vi "ni5660 Configure for IQ.vi"(0 "receiver info in":T1, 1 "acquisition type":string(combo)="FINITE", 5 "carrier frequency (Hz)":dbl=100000000.0 format="%.2p", 7 "bandwidth (Hz)":dbl=20000000.0 format="%.2p", 9 "time duration (sec)":dbl=1e-05 format="%.2p", 11 "error in (no error)":errorcluster, 12 "reference level (dBm)":i32, 13 "auto attenuation":enum16{"DISABLE", "ENABLE"}(ring)=enum."ENABLE", 14 "attenuation (dB)":i32=20) -> (4 "receiver info out":T1, 15 "error out":errorcluster)   [LabVIEW 2011]
doc: "This VI configures the RF Signal Analyzer hardware to acquire a time-domain signal with IQ settings you specify. Carrier frequency, bandwidth, and acquisition time settings define the IQ data. You can configure the acquisition to be finite or continuous. \n\nThis VI configures the reference level and attenuation settings used by the RF downconverter module, and the horizontal settings and acquisition type used by the IF digitizer module."
uses:
  <vilib>/addons/Modulation/niScope/controls/mod_Modulation Settings.ctl
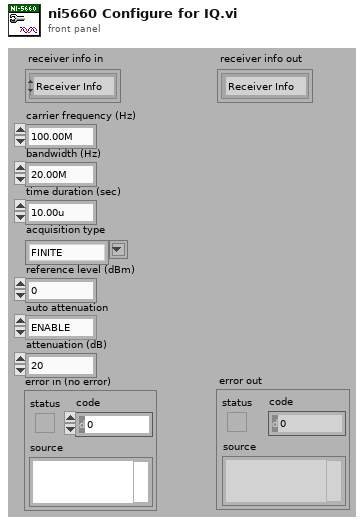
[diagram p1: front panel]
types:
  T1 = typedef "mod_Modulation Settings.ctl" = cluster{enum16{"Receiver Info"}, variant}
  T2 = typedef "mod_Readable Attributes Cluster.ctl" = cluster{"carrier":cluster{"frequency":dbl}, "receiver":cluster{"handles":cluster{"niTuner taskID":i32, "niScope handle":refnum<k15>}, "RFSA":cluster{"reference level":i32, "RF attenuation":i32}, "data format":enum16{"real", "complex modulated (array)", "complex modulated (interleaved)"}, "auto suppress SW IQ":enum16{"off", "on"}, "IQ sample rate":dbl, "bandwidth":dbl}}
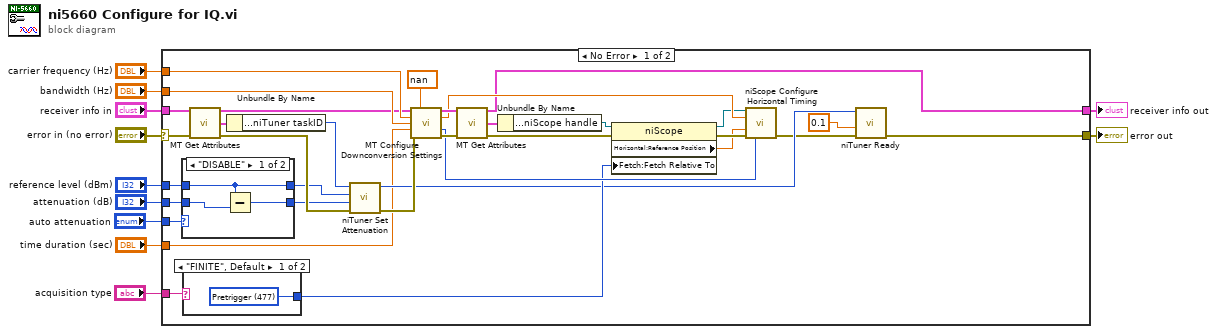
[diagram p0: block diagram]
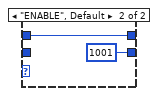
[diagram p2: hidden frame]
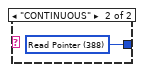
[diagram p3: hidden frame]
diagram:
  n1 = case shown="No Error" "error in (no error)" {
    selector: "error in (no error)" -> [w25 w53]
    tunnel: [w14 w53] -> w11
    tunnel: "carrier frequency (Hz)" -> [w42 _]
    tunnel: "bandwidth (Hz)" -> [w41 _]
    tunnel: "time duration (sec)" -> [w12 _]
    tunnel: "reference level (dBm)" -> [w29 _]
    tunnel: "attenuation (dB)" -> [w28 _]
    tunnel: [w13 w52] -> w1
    tunnel: "receiver info in" -> [w26 w52]
    tunnel: "acquisition type" -> [w31 _]
    tunnel: "auto attenuation" -> [w30 _]
    frame No Error {
      n2 = case shown="\"DISABLE\"" w30 {
        tunnel: [w47 w49] -> w15
        tunnel: w29 -> [w47 w49]
        tunnel: w28 -> [w46 _]
        tunnel: [w45 1001] -> w21
        frame "DISABLE" {
          n3 = Subtract(x=w47, y=w46) -> (x-y=w45:i32)
        }
        frame "ENABLE", Default {
        }
      }
      n4 = case shown="\"FINITE\", Default" w31 {
        tunnel: [w50 w51] -> w32
        frame "FINITE", Default {
          w50 = 477 items=["Start"=482, "Trigger"=483, "Pretrigger"=477, "Now"=481, "Read Pointer"=388] ("Fetch:Fetch Relative To")
        }
        frame "CONTINUOUS" {
          w51 = 388 items=["Start"=482, "Trigger"=483, "Pretrigger"=477, "Now"=481, "Read Pointer"=388] ("Fetch:Fetch Relative To")
        }
      }
      n5 = call <vilib>:"MT Get Attributes.vi"("receiver info in"=w26, "error in (no error)"=w25) -> ("receiver info out"=w22:T1, "attributes"=w27:T2, "error out"=w24:errorcluster)  [unwired: 11 in]
      n6 = Unbundle By Name(w27) -> ("receiver.handles.niTuner taskID"=w20:i32)
      n7 = call <instrlib>:"niTuner Set Attenuation.vi"("error in"=w24, "mixer level (dBm)"=w21, "ref level (dBm)"=w15, "taskID in"=w20) -> ("error out"=w23:errorcluster, "taskID out"=w19:i32)  [unwired: 4 in, 2 out]
      n8 = call <vilib>:"MT Configure Downconversion Settings.vi"("receiver info in"=w22, "min IQ sample rate (S/sec) (NaN:auto)"=nan, "carrier frequency (Hz)"=w42, "bandwidth (Hz)"=w41, "time duration (sec)"=w12, "error in (no error)"=w23) -> ("receiver info out"=w44:T1, "niScope sample rate (S/sec)"=w39:dbl, "number of samples"=w38:i32, "error out"=w43:errorcluster)  [unwired: 6 in]
      n9 = call <vilib>:"MT Get Attributes.vi"("receiver info in"=w44, "error in (no error)"=w43) -> ("receiver info out"=w13:T1, "attributes"=w16:T2, "error out"=w37:errorcluster)  [unwired: 11 in]
      n10 = Unbundle By Name(w16) -> ("receiver.handles.niScope handle"=w36:refnum<k15>)
      n11 = property on="Property Node" class="niScope"(reference=w36, error in=w37, "Fetch:Fetch Relative To"=w32) -> (reference out=w35:refnum<k15>, error out=w34:errorcluster, "Horizontal:Reference Position"=w33:dbl)
      n12 = call <instrlib>:"niScope Configure Horizontal Timing.vi"("instrument handle"=w35, "min sample rate"=w39, "reference position"=w33, "error in"=w34, "min record length"=w38) -> ("error out"=w18:errorcluster)  [unwired: 9 in, 1 out]
      n13 = call <instrlib>:"niTuner Ready.vi"("error in"=w18, "timeout"=0.1, "taskID in"=w19) -> ("error out"=w14:errorcluster)  [unwired: 6 in, 2 out]
    }
    frame Error {
    }
  }
  "error out" <- w11
  "receiver info out" <- w1
